vi "Perform Action.vi"(8 "error in (no error)":errorcluster, 10 "Input":variant, 11 "PWM CFG in":refnum<class "PWM CFG.lvclass">) -> (0 "error out":errorcluster, 2 "Output":variant, 3 "PWM CFG out":refnum<class "PWM CFG.lvclass">)   [LabVIEW 2023, in "DIO Simulated.lvlib" / "PWM CFG.lvclass"]
uses:
  PWM CFG.lvclass
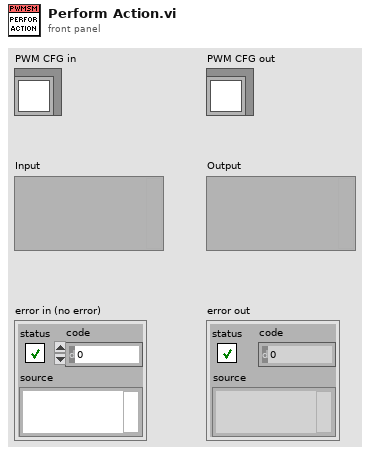
[diagram p1: front panel]
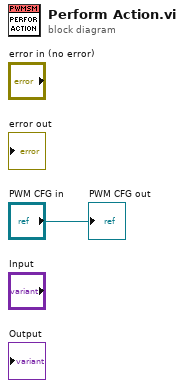
[diagram p0: block diagram]
diagram:
  "PWM CFG out" <- "PWM CFG in"
